vi "niScope Actual Sample Mode.vi"(0 "instrument handle":refnum<k15>, 11 "error in":errorcluster) -> (4 "instrument handle out":refnum<k15>, 8 "sample mode":i32, 15 "error out":errorcluster)   [LabVIEW 2011]
doc: "Returns the sample mode the digitizer is currently using."
uses:
  niScope_32.dll
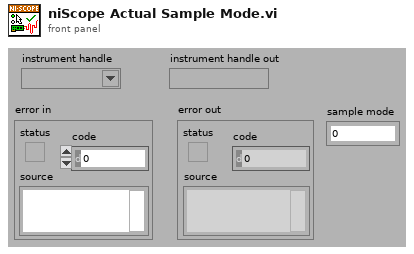
[diagram p1: front panel]
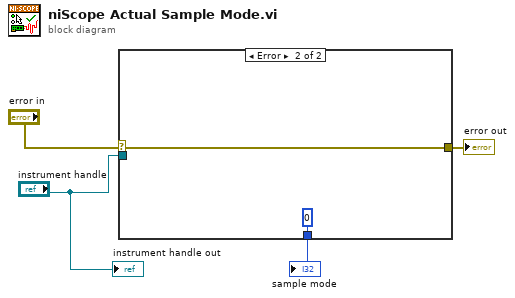
[diagram p0: block diagram]
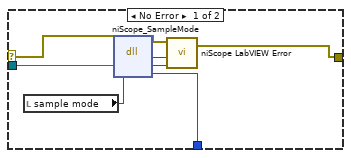
[diagram p2: hidden frame]
diagram:
  n1 = case shown="Error" "error in" {
    selector: "error in" -> [w5 w12]
    tunnel: [w6 w12] -> w4
    tunnel: [w9 0 ("sample mode")] -> w3
    tunnel: "instrument handle" -> [w11 _]
    frame No Error {
      n2 = local read "sample mode"() -> (w10:i32)
      n3 = dll-call lib="niScope_*.*" fn="niScope_SampleMode" ("Call Library Function")("instrument handle"=w11, "sampleMode"=w10) -> ("status"=w7:i32, "instrument handle"=w8:u32, "sampleMode"=w9:i32)  [unwired: 3 in, 2 out]
      n4 = call <instrlib>:"niScope LabVIEW Error.vi"("instrument handle"=w8, "niScope error code (0)"=w7, "error in (no error)"=w5) -> ("error out"=w6:errorcluster)  [unwired: 2 in]
    }
    frame Error {
    }
  }
  "error out" <- w4
  "sample mode" <- w3
  "instrument handle out" <- "instrument handle"
